vi "Write Atts.vi"(6 "Points":i32, 7 "IF_Band":dbl, 8 "error in (no error)":errorcluster, 9 "Stop":dbl, 10 "Start":dbl, 11 "keysight in":refnum<class "keysight.lvclass">) -> (0 "error out":errorcluster, 3 "keysight out":refnum<class "keysight.lvclass">)   [LabVIEW 2015, in "keysight.lvclass"]
uses:
  keysight.lvclass
  keysight.lvclass/keysight.ctl
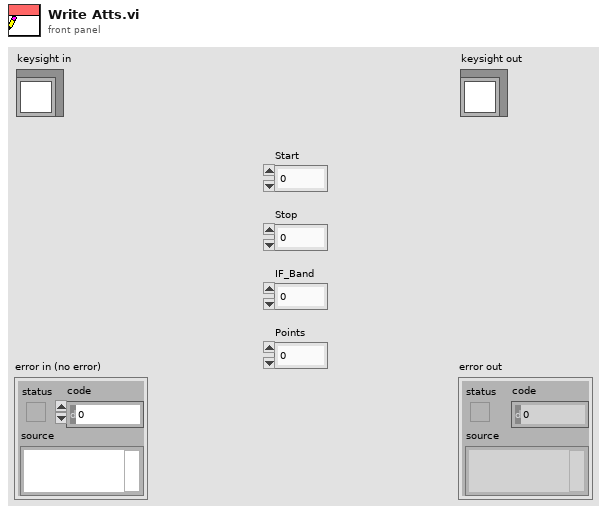
[diagram p1: front panel]
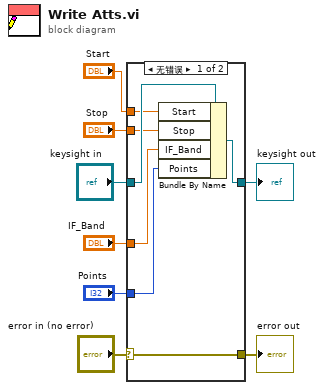
[diagram p0: block diagram]
diagram:
  n1 = case shown="无错误" "error in (no error)" {
    selector: "error in (no error)" -> [w15 w16]
    tunnel: [w15 w16] -> w7
    tunnel: [w9 w17] -> w6
    tunnel: "keysight in" -> [w14 w17]
    tunnel: "Start" -> [w13 _]
    tunnel: "Stop" -> [w12 _]
    tunnel: "IF_Band" -> [w11 _]
    tunnel: "Points" -> [w10 _]
    frame No Error {
      n2 = Bundle By Name(cluster=w14, "Start"=w13, "Stop"=w12, "IF_Band"=w11, "Points"=w10) -> (w9:refnum<class "keysight.lvclass">)
    }
    frame Error {
    }
  }
  "error out" <- w7
  "keysight out" <- w6
